vi "Save Notebook Before Opening One.vi"(2 "Not saved?":bool) -> (7 "Save?":bool)   [LabVIEW 2019, in "Notebook.lvlib"]
uses:
  Notebook.lvlib
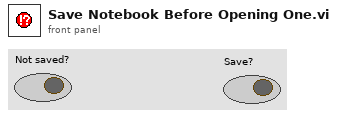
[diagram p1: front panel]
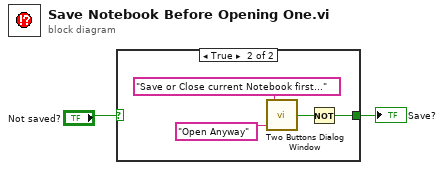
[diagram p0: block diagram]
diagram:
  n1 = case shown="True" "Not saved?" {
    selector: "Not saved?" -> [w3 _]
    tunnel: [w3 w4] -> w1
    frame False {
    }
    frame True {
      n2 = call "Two Buttons Dialog Window.vi"("Cancel Button Text"="Open Anyway" ("F button name (\"Cancel\")"), "Message"="Save or Close current Notebook first..." ("message")) -> ("OK?"=w5:bool)  [unwired: 1 in]
      n3 = Not(x=w5) -> (.not. x?=w4:bool)
    }
  }
  "Save?" <- w1
